vi "Test.vi"() -> ()   [LabVIEW 2015, in "Timer.lvclass"]
uses:
  Timer.lvclass
  <vilib>/Platform/TimedLoop/XDataNode/timing_clust.ctl
  <vilib>/Platform/TimedLoop/XDataNode/nitl_modes.ctl
  <vilib>/Platform/TimedLoop/XDataNode/wakeup.ctl
  Timer.lvclass/Timer.ctl
  <vilib>/platform/TimedLoop/XDataNode/XDataNode.xnode
  <vilib>/Platform/TimedLoop/XDataNode/XDNodeRunTimeDep.lvlib
panel:
  out "Period [s] 2":dbl format="%.4p"
  out "Elapsed Time [s] 2":dbl
  in  "y 2":dbl
  out "Elapsed Time [s]":dbl
  out "Period [s]":dbl format="%.4p"
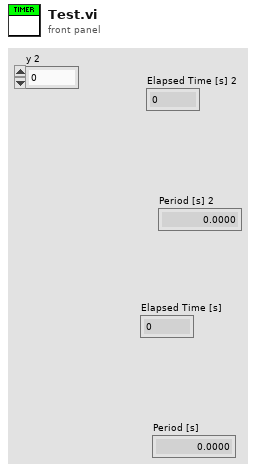
[diagram p1: front panel]
types:
  T1 = typedef "XDNodeRunTimeDep.lvlib/timing_clust.ctl" = cluster{"Expected End [f-1]":u64, "Actual End [f-1]":u64, "Finished Late? [f-1]":bool, "Expected End [i-1]":u64, "Actual End [i-1]":u64, "Finished Late? [i-1]":bool, "Expected Start [i]":u64, "Actual Start [i]":u64, "Expected Start [f]":u64, "Actual Start [f]":u64, "Source Name":string, "Structure Name":string, "Period":i64, "Deadline":i64, "Offset":i64, "Start":i64, "Priority":i32, "Timeout":i32, "Mode":T2, "Wakeup Reason":T3, "Error":errorcluster, "Source Type":string, "Secondary Source Type":string, "Global End Time":u64, "Global Start Time":u64, "Frame Duration":u64, "Iteration Duration":u64, "Assigned CPU":i32, "I/O Scan Engine Mode":u32}
  T2 = typedef "XDNodeRunTimeDep.lvlib/nitl_modes.ctl" = enum32{"No Change", "Process missed periods, maintain original phase", "Discard missed periods, maintain original phase", "Process missed periods, ignore original phase", "Discard missed periods, ignore original phase"}
  T3 = typedef "XDNodeRunTimeDep.lvlib/wakeup.ctl" = enum32{"Normal", "Aborted", "Asynchronous wakeup", "Timing source error", "Timed loop error", "Timeout"}
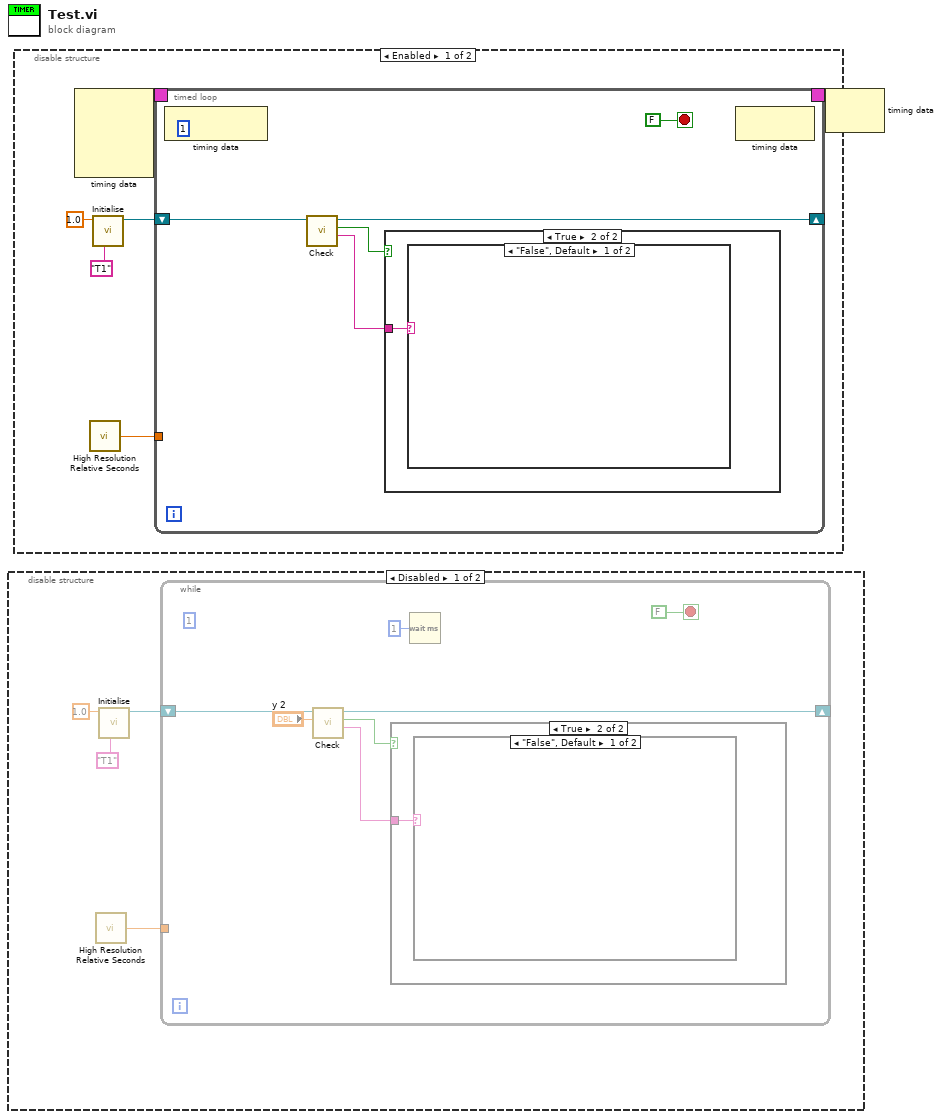
[diagram p0: block diagram]
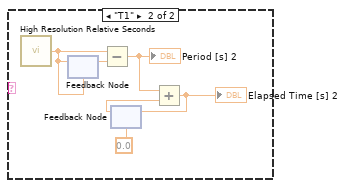
[diagram p3: hidden frame]
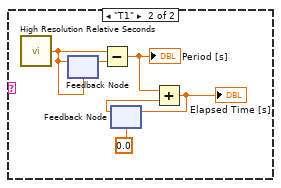
[diagram p6: hidden frame]
diagram:
  n1 = disable-structure shown="Disabled" {
    frame Disabled {
      n2 = call <vilib>:"High Resolution Relative Seconds.vi"() -> ("relative seconds"=w4:dbl)
      n3 = call "Initialise.vi"("Name"="T1", "Period [s]"=1.0) -> ("Timer out"=w3:refnum<class "Timer.lvclass">)  [unwired: 9 in]
      n4 = while {
        shift-right: [w10] -> _
        shift-left: w3 -> [w11]
        tunnel: w4 -> [_]
        stop <- FALSE stop-if-true
        (unwired) 1
        n5 = call "Check.vi"(10:"y 2", "Timer in"=w11) -> ("Name"=w8:string, "Elapsed"=w9:bool, "Timer out"=w10:refnum<class "Timer.lvclass">)  [unwired: 6 in, 1 out]
        n6 = case shown="True" w9 {
          tunnel: w8 -> [_ w12]
          frame False {
          }
          frame True {
            n7 = case shown="\"False\", Default" w12 {
              frame "False", Default {
              }
              frame "T1" {
                n8 = call <vilib>:"High Resolution Relative Seconds.vi"() -> ("relative seconds"=w13:dbl)
                n9 = feedback-in #1(w13) -> ()
                n10 = feedback #1(w13) -> (w18:dbl)
                n11 = Subtract(x=w13, y=w18) -> (x-y=w17:dbl)
                "Period [s] 2" <- w17
                n12 = feedback #2(0.0) -> (w15:dbl)
                n13 = Add(x=w17, y=w15) -> (x+y=w16:dbl)
                "Elapsed Time [s] 2" <- w16
                n14 = feedback-in #2(w16) -> ()
              }
            }
          }
        }
        n15 = Wait (ms)(milliseconds to wait=u32 1) -> ()  [unwired: 1 out]
      }
    }
    frame Enabled {
    }
  }
  n16 = disable-structure shown="Enabled" {
    frame Enabled {
      n17 = node-c288() -> (w24:T1)  [unwired: 4 in]
      n18 = call <vilib>:"High Resolution Relative Seconds.vi"() -> ("relative seconds"=w19:dbl)
      n19 = call "Initialise.vi"("Name"="T1", "Period [s]"=1.0) -> ("Timer out"=w20:refnum<class "Timer.lvclass">)  [unwired: 9 in]
      n20 = timed-loop {
        shift-right: [w28] -> _
        shift-left: w20 -> [w29]
        timing: w24 -> [_]
        timing-out: [_] -> w23
        tunnel: w19 -> [_]
        stop <- FALSE stop-if-true
        (unwired) 1
        n21 = node-c288() -> ()  [unwired: 1 in, 1 out]
        n22 = call "Check.vi"("Timer in"=w29) -> ("Name"=w26:string, "Elapsed"=w27:bool, "Timer out"=w28:refnum<class "Timer.lvclass">)  [unwired: 7 in, 1 out]
        n23 = case shown="True" w27 {
          tunnel: w26 -> [_ w30]
          frame False {
          }
          frame True {
            n24 = case shown="\"False\", Default" w30 {
              frame "False", Default {
              }
              frame "T1" {
                n25 = call <vilib>:"High Resolution Relative Seconds.vi"() -> ("relative seconds"=w31:dbl)
                n26 = feedback-in #3(w31) -> ()
                n27 = feedback #3(w31) -> (w36:dbl)
                n28 = Subtract(x=w31, y=w36) -> (x-y=w35:dbl)
                "Period [s]" <- w35
                n29 = feedback #4(0.0) -> (w33:dbl)
                n30 = Add(x=w35, y=w33) -> (x+y=w34:dbl)
                "Elapsed Time [s]" <- w34
                n31 = feedback-in #4(w34) -> ()
              }
            }
          }
        }
        n32 = node-c288() -> ()  [unwired: 1 in, 1 out]
      }
      n33 = node-c288(w23) -> ()  [unwired: 1 out]
    }
    frame Disabled {
    }
  }
